vi "customTransferFunction.vi"(1 "Denominator":T1={"d2"=-5.379109252820069, "d3"=13.338745817780108, "d4"=-19.871028145479414, "d5"=19.50746353229121, "d6"=-13.043244632828106, "d7"=5.924549706009071, "d8"=-1.7592519447216297, "d9"=0.3093734613503629, "d10"=-0.024514322011746192} {"d10" format="%#_54g"; "d9" format="%#_52g"; "d8" format="%#_49g"; "d7" format="%#_49g"; "d6" format="%#_47g"; "d5" format="%#_47g"; "d4" format="%#_47g"; "d3" format="%#_47g"; "d2" format="%#_50g"}, 2 "Numerator":T2={"n2"=0.779209781450863, "n3"=-4.478196131314931, "n4"=12.236859326708696, "n5"=-20.5353561507535, "n6"=23.027520703445788, "n7"=-17.63415125244481, "n8"=9.00853418240981, "n9"=-2.8149211692703915, "n10"=0.41348492933818193} {"n10" format="%#_52g"; "n9" format="%#_51g"; "n8" format="%#_51g"; "n7" format="%#_51g"; "n6" format="%#_51g"; "n5" format="%#_51g"; "n4" format="%#_51g"; "n3" format="%#_51g"; "n2" format="%#_51g"}, 3 "x[k]":fxp<+/-,32,8>, 4 "reset":bool) -> (0 "y[k]":fxp<+/-,40,16> format="%#_15g")   [LabVIEW 2020]
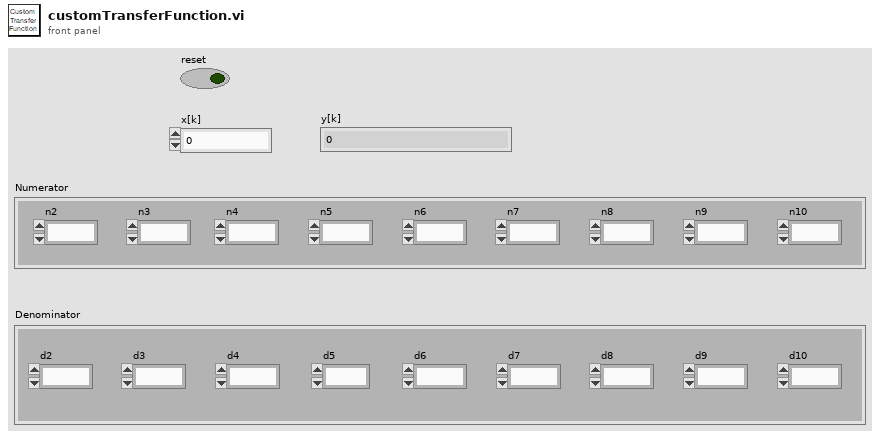
[diagram p1: front panel]
types:
  T1 = cluster{"d2":fxp<+/-,52,4>, "d3":fxp<+,49,4>, "d4":fxp<+/-,51,6>, "d5":fxp<+,50,5>, "d6":fxp<+/-,50,5>, "d7":fxp<+,51,3>, "d8":fxp<+/-,50,2>, "d9":fxp<+,51,-1>, "d10":fxp<+/-,51,-4>}
  T2 = cluster{"n2":fxp<+,51,0>, "n3":fxp<+/-,52,4>, "n4":fxp<+,49,4>, "n5":fxp<+/-,51,6>, "n6":fxp<+,50,5>, "n7":fxp<+/-,51,6>, "n8":fxp<+,52,4>, "n9":fxp<+/-,51,3>, "n10":fxp<+,51,-1>}
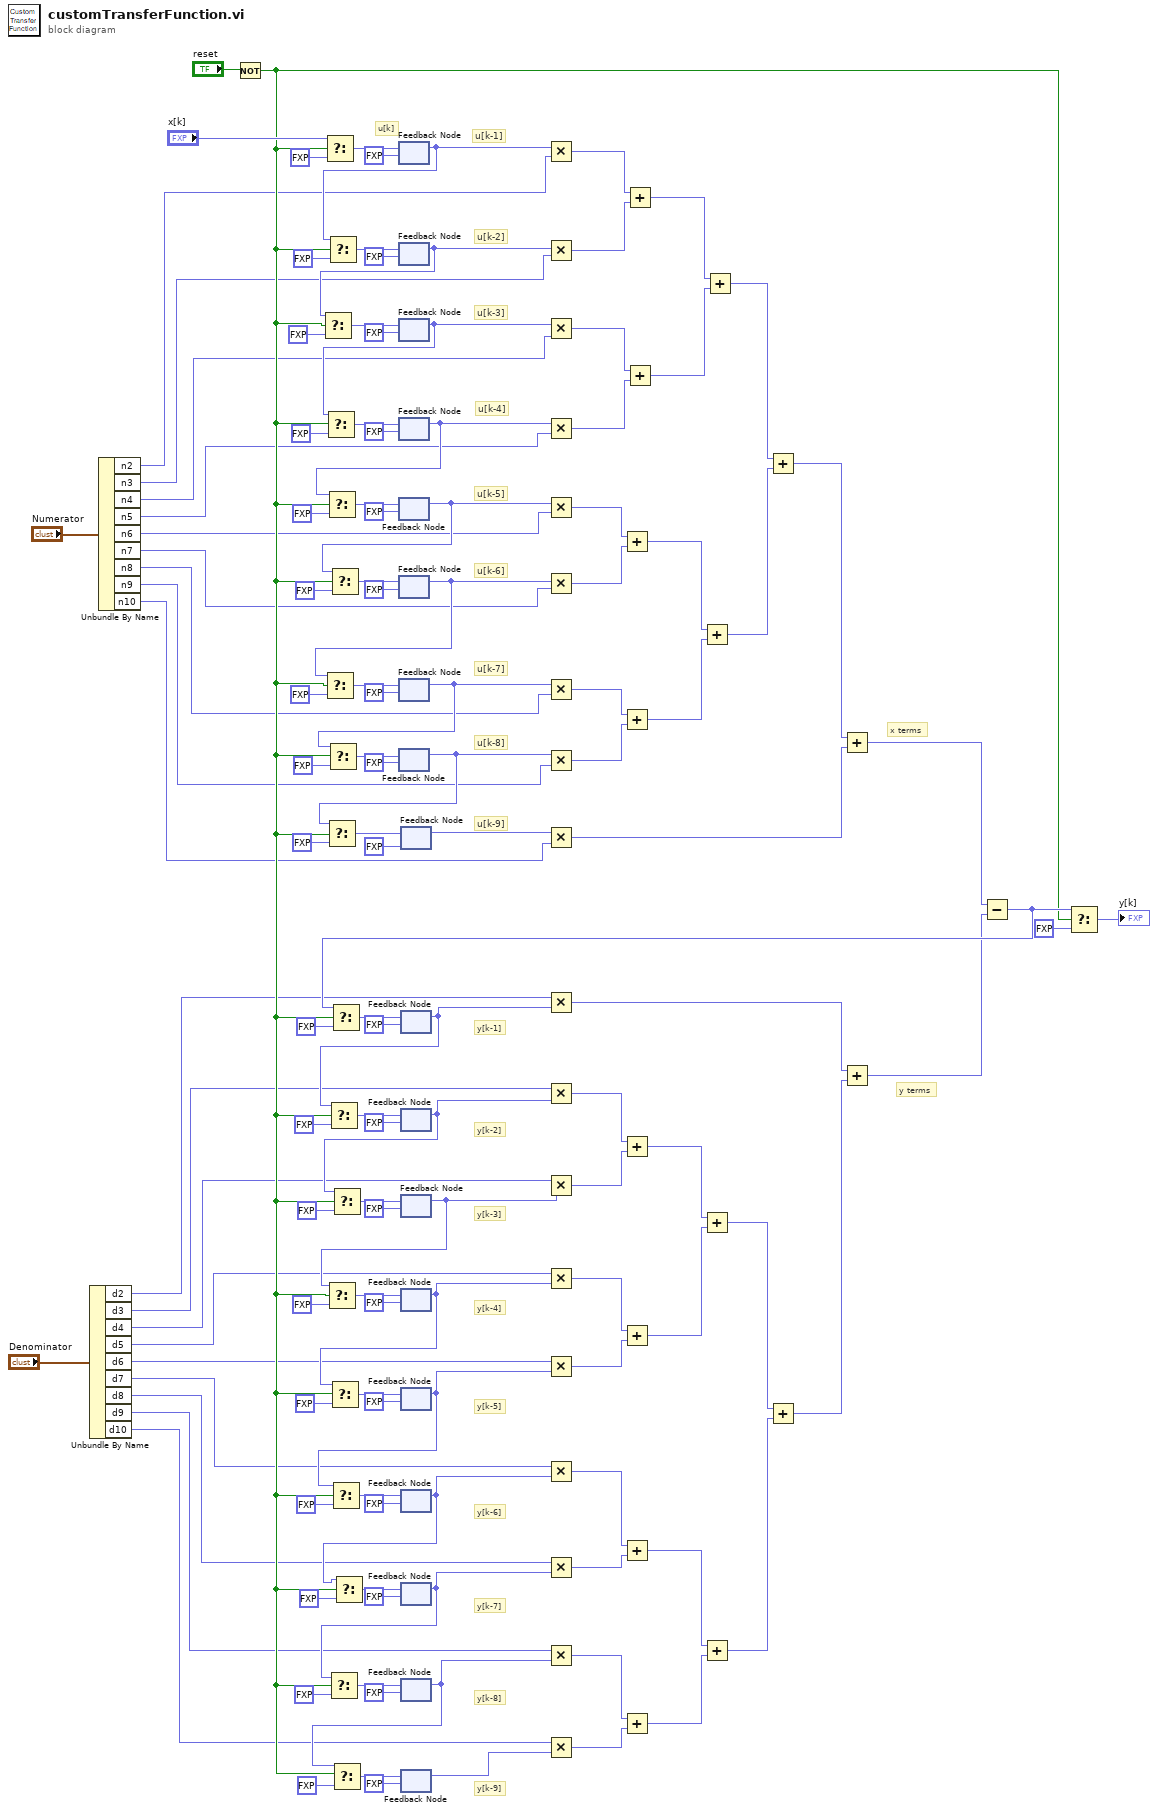
[diagram p0: block diagram]
diagram:
  # "y terms"
  # "x terms"
  # "y[k-9]"
  # "y[k-8]"
  # "y[k-7]"
  # "y[k-6]"
  # "y[k-5]"
  # "y[k-4]"
  # "y[k-3]"
  # "u[k-9]"
  # "u[k-8]"
  # "u[k-7]"
  # "u[k-6]"
  # "u[k-5]"
  # "u[k-4]"
  # "u[k-3]"
  # "u[k-2]"
  # "u[k]"
  # "y[k-2]"
  # "y[k-1]"
  # "u[k-1]"
  n1 = Unbundle By Name("Denominator") -> ("d2"=w9:fxp<+/-,52,4>, "d3"=w8:fxp<+,49,4>, "d4"=w7:fxp<+/-,51,6>, "d5"=w1:fxp<+,50,5>, "d6"=w6:fxp<+/-,50,5>, "d7"=w5:fxp<+,51,3>, "d8"=w4:fxp<+/-,50,2>, "d9"=w3:fxp<+,51,-1>, "d10"=w2:fxp<+/-,51,-4>)
  n2 = Unbundle By Name("Numerator") -> ("n2"=w19:fxp<+,51,0>, "n3"=w18:fxp<+/-,52,4>, "n4"=w17:fxp<+,49,4>, "n5"=w16:fxp<+/-,51,6>, "n6"=w15:fxp<+,50,5>, "n7"=w14:fxp<+/-,51,6>, "n8"=w13:fxp<+,52,4>, "n9"=w12:fxp<+/-,51,3>, "n10"=w11:fxp<+,51,-1>)
  n3 = Not(x="reset") -> (.not. x?=w31:bool)
  n4 = Select(t="x[k]", s=w31, f=fxp<+/-,32,8> 0.0 ("u[k]")) -> (s? t:f=w86:fxp<+/-,32,8>)
  n5 = feedback #1(fxp<+/-,32,8> 0.0 ("u[k]")) -> (w81:fxp<+/-,32,8>)
  n6 = Select(t=w81, s=w31, f=fxp<+/-,32,8> 0.0 ("u[k]")) -> (s? t:f=w80:fxp<+/-,32,8>)
  n7 = feedback-in #1(w86) -> ()
  n8 = feedback #2(fxp<+/-,32,8> 0.0 ("u[k]")) -> (w77:fxp<+/-,32,8>)
  n9 = Select(t=w77, s=w31, f=fxp<+/-,32,8> 0.0 ("u[k]")) -> (s? t:f=w76:fxp<+/-,32,8>)
  n10 = feedback-in #2(w80) -> ()
  n11 = feedback #3(fxp<+/-,32,8> 0.0 ("u[k]")) -> (w75:fxp<+/-,32,8>)
  n12 = Select(t=w75, s=w31, f=fxp<+/-,32,8> 0.0 ("u[k]")) -> (s? t:f=w74:fxp<+/-,32,8>)
  n13 = feedback-in #3(w76) -> ()
  n14 = feedback #4(fxp<+/-,32,8> 0.0 ("u[k]")) -> (w69:fxp<+/-,32,8>)
  n15 = Select(t=w69, s=w31, f=fxp<+/-,32,8> 0.0 ("u[k]")) -> (s? t:f=w68:fxp<+/-,32,8>)
  n16 = feedback-in #4(w74) -> ()
  n17 = feedback #5(fxp<+/-,32,8> 0.0 ("u[k]")) -> (w67:fxp<+/-,32,8>)
  n18 = Select(t=w67, s=w31, f=fxp<+/-,32,8> 0.0 ("u[k]")) -> (s? t:f=w66:fxp<+/-,32,8>)
  n19 = feedback-in #5(w68) -> ()
  n20 = feedback #6(fxp<+/-,32,8> 0.0 ("u[k]")) -> (w65:fxp<+/-,32,8>)
  n21 = Select(t=w65, s=w31, f=fxp<+/-,32,8> 0.0 ("u[k]")) -> (s? t:f=w64:fxp<+/-,32,8>)
  n22 = feedback-in #6(w66) -> ()
  n23 = feedback #7(fxp<+/-,32,8> 0.0 ("u[k]")) -> (w62:fxp<+/-,32,8>)
  n24 = Select(t=w62, s=w31, f=fxp<+/-,32,8> 0.0 ("u[k]")) -> (s? t:f=w61:fxp<+/-,32,8>)
  n25 = feedback-in #7(w64) -> ()
  n26 = feedback #8(fxp<+/-,32,8> 0.0 ("u[k]")) -> (w60:fxp<+/-,32,8>)
  n27 = Select(t=w60, s=w31, f=fxp<+/-,32,8> 0.0 ("u[k]")) -> (s? t:f=w59:fxp<+/-,32,8>)
  n28 = feedback-in #8(w61) -> ()
  n29 = feedback #9(fxp<+/-,32,8> 0.0 ("u[k]")) -> (w114:fxp<+/-,32,8>)
  n30 = feedback-in #9(w59) -> ()
  n31 = feedback #10(fxp<+/-,40,16> 0.0) -> (w47:fxp<+/-,40,16>)
  n32 = Select(t=w47, s=w31, f=fxp<+/-,32,8> 0.0 ("u[k]")) -> (s? t:f=w46:fxp<+/-,40,16>)
  n33 = feedback #11(fxp<+/-,40,16> 0.0) -> (w44:fxp<+/-,40,16>)
  n34 = Select(t=w44, s=w31, f=fxp<+/-,32,8> 0.0 ("u[k]")) -> (s? t:f=w45:fxp<+/-,40,16>)
  n35 = feedback-in #11(w46) -> ()
  n36 = feedback #12(fxp<+/-,40,16> 0.0) -> (w42:fxp<+/-,40,16>)
  n37 = Select(t=w42, s=w31, f=fxp<+/-,32,8> 0.0 ("u[k]")) -> (s? t:f=w43:fxp<+/-,40,16>)
  n38 = feedback-in #12(w45) -> ()
  n39 = feedback #13(fxp<+/-,40,16> 0.0) -> (w40:fxp<+/-,40,16>)
  n40 = Select(t=w40, s=w31, f=fxp<+/-,32,8> 0.0 ("u[k]")) -> (s? t:f=w41:fxp<+/-,40,16>)
  n41 = feedback-in #13(w43) -> ()
  n42 = feedback #14(fxp<+/-,40,16> 0.0) -> (w38:fxp<+/-,40,16>)
  n43 = Select(t=w38, s=w31, f=fxp<+/-,32,8> 0.0 ("u[k]")) -> (s? t:f=w39:fxp<+/-,40,16>)
  n44 = feedback-in #14(w41) -> ()
  n45 = feedback #15(fxp<+/-,40,16> 0.0) -> (w36:fxp<+/-,40,16>)
  n46 = Select(t=w36, s=w31, f=fxp<+/-,32,8> 0.0 ("u[k]")) -> (s? t:f=w37:fxp<+/-,40,16>)
  n47 = feedback-in #15(w39) -> ()
  n48 = feedback #16(fxp<+/-,40,16> 0.0) -> (w33:fxp<+/-,40,16>)
  n49 = Select(t=w33, s=w31, f=fxp<+/-,32,8> 0.0 ("u[k]")) -> (s? t:f=w32:fxp<+/-,40,16>)
  n50 = feedback-in #16(w37) -> ()
  n51 = feedback #17(fxp<+/-,40,16> 0.0) -> (w34:fxp<+/-,40,16>)
  n52 = Select(t=w34, s=w31, f=fxp<+/-,32,8> 0.0 ("u[k]")) -> (s? t:f=w35:fxp<+/-,40,16>)
  n53 = feedback-in #17(w32) -> ()
  n54 = feedback #18(fxp<+/-,40,16> 0.0) -> (w113:fxp<+/-,40,16>)
  n55 = feedback-in #18(w35) -> ()
  n56 = Multiply(x=w81, y=w19) -> (x*y=w112:fxp<+/-,32,8>)
  n57 = Multiply(x=w77, y=w18) -> (x*y=w111:fxp<+/-,34,10>)
  n58 = Multiply(x=w75, y=w17) -> (x*y=w110:fxp<+/-,36,12>)
  n59 = Multiply(x=w69, y=w16) -> (x*y=w109:fxp<+/-,36,12>)
  n60 = Multiply(x=w67, y=w15) -> (x*y=w108:fxp<+/-,37,13>)
  n61 = Multiply(x=w65, y=w14) -> (x*y=w107:fxp<+/-,36,12>)
  n62 = Multiply(x=w62, y=w13) -> (x*y=w106:fxp<+/-,35,11>)
  n63 = Multiply(x=w60, y=w12) -> (x*y=w105:fxp<+/-,34,10>)
  n64 = Multiply(x=w114, y=w11) -> (x*y=w104:fxp<+/-,32,7>)
  n65 = Multiply(x=w9, y=w47) -> (x*y=w103:fxp<+/-,35,11>)
  n66 = Multiply(x=w8, y=w44) -> (x*y=w102:fxp<+/-,37,13>)
  n67 = Multiply(x=w7, y=w42) -> (x*y=w101:fxp<+/-,37,13>)
  n68 = Multiply(x=w1, y=w40) -> (x*y=w100:fxp<+/-,37,13>)
  n69 = Multiply(x=w6, y=w38) -> (x*y=w99:fxp<+/-,37,13>)
  n70 = Multiply(x=w5, y=w36) -> (x*y=w98:fxp<+/-,35,11>)
  n71 = Multiply(x=w4, y=w33) -> (x*y=w97:fxp<+/-,34,10>)
  n72 = Multiply(x=w3, y=w34) -> (x*y=w96:fxp<+/-,32,7>)
  n73 = Multiply(x=w2, y=w113) -> (x*y=w95:fxp<+/-,32,4>)
  n74 = Add(x=w108, y=w107) -> (x+y=w92:fxp<+/-,37,13>)
  n75 = Add(x=w106, y=w105) -> (x+y=w91:fxp<+/-,36,12>)
  n76 = Add(x=w102, y=w101) -> (x+y=w87:fxp<+/-,38,14>)
  n77 = Add(x=w100, y=w99) -> (x+y=w88:fxp<+/-,38,14>)
  n78 = Add(x=w98, y=w97) -> (x+y=w90:fxp<+/-,36,12>)
  n79 = Add(x=w96, y=w95) -> (x+y=w89:fxp<+/-,32,7>)
  n80 = Add(x=w112, y=w111) -> (x+y=w94:fxp<+/-,34,10>)
  n81 = Add(x=w110, y=w109) -> (x+y=w93:fxp<+/-,37,13>)
  n82 = Add(x=w92, y=w91) -> (x+y=w29:fxp<+/-,38,14>)
  n83 = Add(x=w87, y=w88) -> (x+y=w24:fxp<+/-,39,15>)
  n84 = Add(x=w90, y=w89) -> (x+y=w23:fxp<+/-,36,12>)
  n85 = Add(x=w94, y=w93) -> (x+y=w30:fxp<+/-,37,13>)
  n86 = Add(x=w30, y=w29) -> (x+y=w28:fxp<+/-,39,15>)
  n87 = Add(x=w24, y=w23) -> (x+y=w25:fxp<+/-,39,15>)
  n88 = Add(x=w28, y=w104) -> (x+y=w26:fxp<+/-,39,15>)
  n89 = Add(x=w103, y=w25) -> (x+y=w27:fxp<+/-,39,15>)
  n90 = Subtract(x=w26, y=w27) -> (x-y=w49:fxp<+/-,40,16>)
  n91 = Select(t=w49, s=w31, f=fxp<+/-,32,8> 0.0 ("u[k]")) -> (s? t:f=w48:fxp<+/-,40,16>)
  n92 = feedback-in #10(w48) -> ()
  n93 = Select(t=w49, s=w31, f=fxp<+/-,32,8> 0.0 ("u[k]")) -> (s? t:f=→"y[k]":fxp<+/-,40,16>)
